vi "Student t Moments.vi"(10 "k degrees of freedom":i32=1) -> (0 "error":i32, 2 "variance":dbl=1.0, 3 "mean":dbl)   [LabVIEW 2020, in "NI_Gmath.lvlib"]
doc: "Returns the expected mean and variance of the random variate X, where X describes the selected distribution type. You must manually select the polymorphic instance to use."
uses:
  <vilib>/gmath/NI_Gmath.lvlib
  <vilib>/gmath/statdist.llb/st_error_code.ctl
panel:
  # "Student t Moments"
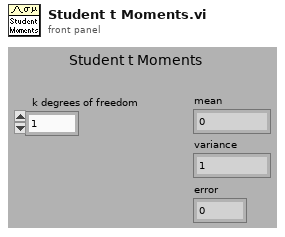
[diagram p1: front panel]
types:
  T1 = typedef "NI_Gmath.lvlib/st_error_code.ctl" = i32
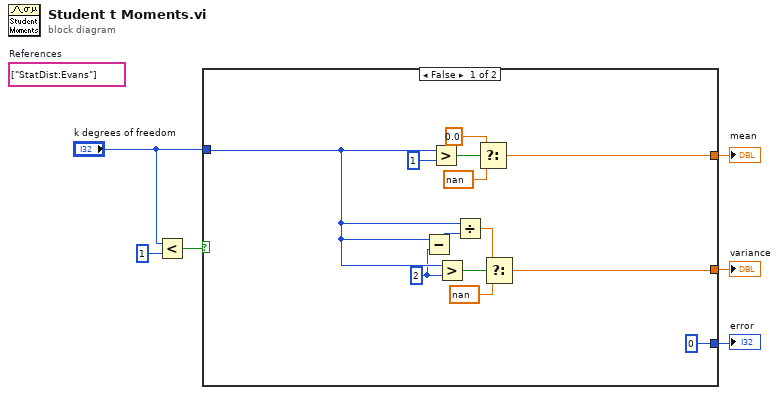
[diagram p0: block diagram]
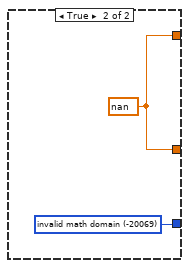
[diagram p2: hidden frame]
diagram:
  (unwired) string[] ["StatDist:Evans"]  # References
  n1 = Less?(x="k degrees of freedom", y=1) -> (x < y?=w2:bool)
  n2 = case shown="False" w2 {
    tunnel: [0 ("invalid math domain") w20] -> w6
    tunnel: [w14 w21] -> w5
    tunnel: "k degrees of freedom" -> [w8 _]
    tunnel: [w11 w21] -> w1
    frame False {
      w7 = 2 ("y")
      n3 = Subtract(x=w8, y=w7) -> (x-y=w9:i32)
      n4 = Greater?(x=w8, y=1) -> (0:w17:bool)
      n5 = Greater?(x=w8, y=w7) -> (0:w12:bool)
      n6 = Divide(x=w8, y=w9) -> (x/y=w10:dbl)
      n7 = Select(t=0.0, s=w17, f=nan) -> (s? t:f=w14:dbl)
      n8 = Select(t=w10, s=w12, f=nan) -> (s? t:f=w11:dbl)
    }
    frame True {
      w20 = T1 -20069 items=["invalid math domain"=-20069, "Fourier interpolation size m >= n"=-20070, "empty array"=-20003] ("stat interp error code")
      w21 = nan
    }
  }
  "mean" <- w5
  "error" <- w6
  "variance" <- w1
